vi "__Local List DoubleClick Handler.vi"(8 "error in (no error)":errorcluster, 10 "Clicked Row":i32, 11 "FileManager Data in":T1) -> (0 "error out":errorcluster, 3 "FileManager Data out":T1)   [LabVIEW 2011]
doc: "This VI handles the double-click on the Local list.\nIf the selected item is a folder, its contents will be listed. Basically this VI is responsible for navigating in the local file system."
uses:
  __File manager Data type.ctl
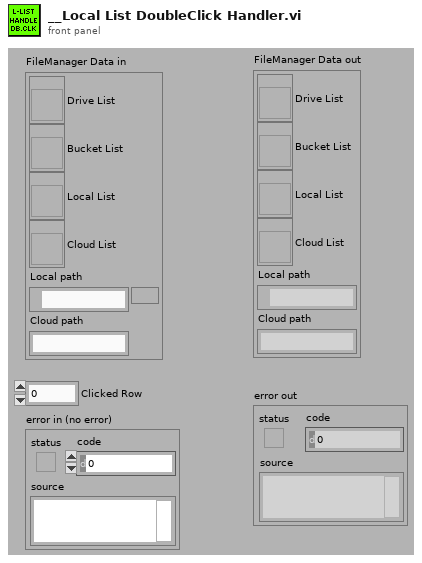
[diagram p1: front panel]
types:
  T1 = typedef "__File manager Data type.ctl" = cluster{"Drive List":refnum<vi>, "Bucket List":refnum<vi>, "Local List":refnum<vi>, "Cloud List":refnum<vi>, "Local path":path, "Cloud path":string}
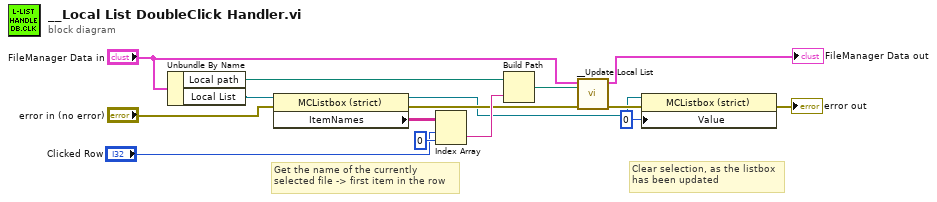
[diagram p0: block diagram]
diagram:
  # "Clear selection, as the listbox\nhas been updated"
  # "Get the name of the currently\nselected file -> first item in the row"
  n1 = Unbundle By Name("FileManager Data in") -> ("Local path"=w13:path, "Local List"=w1:refnum<vi>)
  n2 = property class="MCListbox (strict)"(reference=w1, error in="error in (no error)") -> (reference out=w6:refnum<vi>, error out=w11:errorcluster, "ItemNames"=w15:string[][])
  n3 = Index Array(array=w15, index (row)="Clicked Row", index (col)=0 ("disabled index (col)")) -> (element=w12:string)
  n4 = Build Path(base path=w13, name or relative path=w12) -> (appended path=w10:path)
  n5 = call "__Update Local List.vi"("error in (no error)"=w11, "Path to list"=w10, "FileManager Ctl Refs in"="FileManager Data in") -> ("error out"=w7:errorcluster, "FileManager Ctl Refs out"=→"FileManager Data out":T1)  [unwired: 7 in]
  n6 = property class="MCListbox (strict)"(reference=w6, error in=w7, "Value"=0) -> (error out=→"error out":errorcluster)  [unwired: 1 out]
